vi "Extract Value.vi"(7 "Raw Data Waveform":T1, 8 "Error":errorcluster, 11 "(Index_Pointer)":refnum<class "Index_Pointer.lvclass">) -> (0 "Error Out":errorcluster, 2 "Value Out":dbl, 3 "(Index_Pointer) Out":refnum<class "Index_Pointer.lvclass">, 5 "Buffer Out":T1)   [LabVIEW 2025, in "Index_Pointer.lvclass"]
uses:
  Index_Pointer.lvclass
  Universal Controls/Waveform_Data.ctl
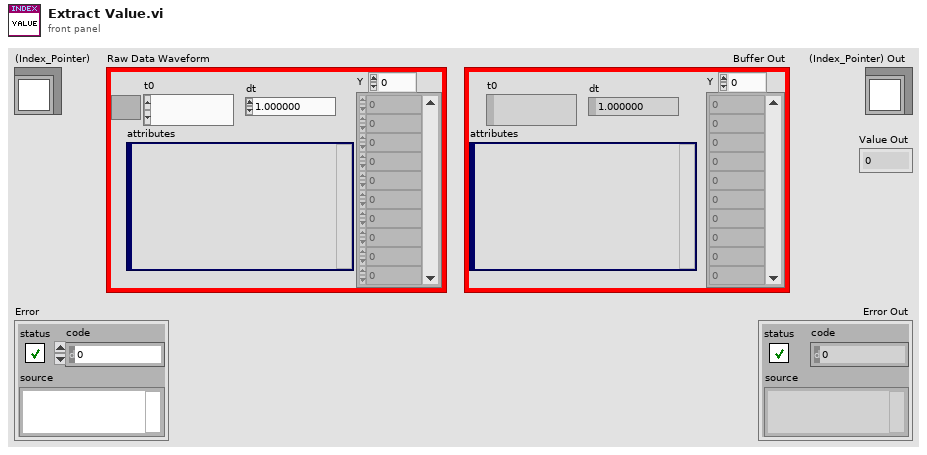
[diagram p1: front panel]
types:
  T1 = typedef "Waveform_Data.ctl" = waveform(dbl)
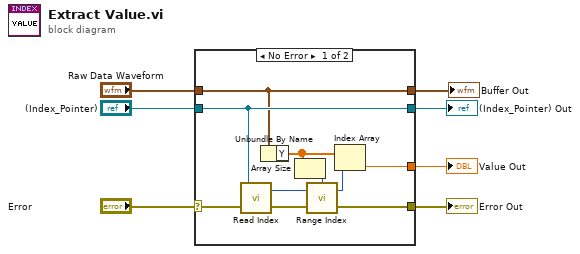
[diagram p0: block diagram]
diagram:
  n1 = case shown="No Error" "Error" {
    selector: "Error" -> [w15 w18]
    tunnel: [w15 w18] -> w4
    tunnel: [w14 w17] -> w6
    tunnel: "(Index_Pointer)" -> [w14 w17]
    tunnel: "Raw Data Waveform" -> [w8 w16]
    tunnel: [w13 _] -> w2
    tunnel: [w8 w16] -> w1
    frame No Error {
      n2 = call "Read Index.vi"("Index_Pointer)"=w14) -> ("Index Out"=w11:i32)  [unwired: 2 in]
      n3 = Unbundle By Name(w8) -> ("Y"=w12:dbl[])
      n4 = Array Size(array=w12) -> (size(s)=w10:i32)
      n5 = call "Range Index.vi"("Index"=w11, "Size"=w10) -> ("Index Out Out"=w9:i32)  [unwired: 1 in]
      n6 = Index Array(array=w12, index=w9) -> (element=w13:dbl)
    }
    frame Error {
    }
  }
  "(Index_Pointer) Out" <- w6
  "Error Out" <- w4
  "Value Out" <- w2
  "Buffer Out" <- w1
